vi "xiLIB - PRM_Limit.vi"(4 "PRM":T2=enum."DEVICE_NAME", 6 "Type":T1, 8 "error in (no error)":errorcluster, 9 "Ctl Refnum":refnum<vi>, 11 "xiCam In":refnum<k24>) -> (0 "error out":errorcluster, 3 "xiCam Out":refnum<k24>)   [LabVIEW 2015]
uses:
  C:/GIT/Cameras3.x/Integrations/Labview/xiLib/xiLIB_32bit/xiLIB/xiCamLib/API/x86/xiApi.NET.dll
  xiLIB_32bit/xiLIB/xiCamLib/API/x86/xiApi.NET.dll
  Typedefs/xiLIB - PRM_Type.ctl
  xiCam/PRM/PRM/PRM_v2.ctl
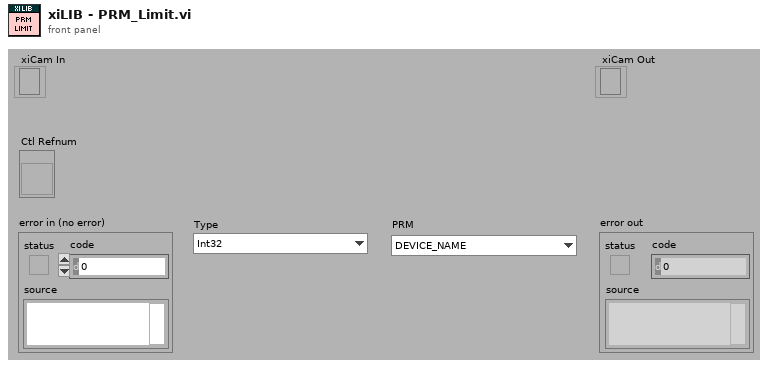
[diagram p1: front panel]
types:
  T1 = typedef "xiLIB - PRM_Type.ctl" = enum16{"Int32", "Float", "String", "DOWNSAMPLING_TYPE", "IMAGE_DATA_FORMAT", "BUFFER_POLICY", "TRG_SOURCE", "GPI", "GPO", "ACQ_TIMING_MODE", "BINNING_PATTERN", "BINNING_SELECTOR", "CMS_MODE", "COUNTER_SELECTOR", "DEBUG_LEVEL", "DECIMATION_PATTERN", "DECIMATION_SELECTOR", "GAIN_SELECTOR_TYPE", "LED_MODE", "LENS_FEATURE_SELECTOR", "LENS_MODE", "OUTPUT_DATA_PACKING_TYPE", "SENSOR_FEATURE_SELECTOR", "SHUTTER_TYPE", "TRG_SELECTOR", "TS_RST_MODE", "TS_RST_SOURCE"}
  T2 = typedef "PRM_v2.ctl" = enum16{"ACQ_BUFFER_SIZE", "ACQ_FRAME_BURST_COUNT", "ACQ_TIMING_MODE", "ACQ_TRANSPORT_BUFFER_SIZE", "AE_MAX_LIMIT", "AEAG", "AEAG_LEVEL", "API_VERSION", "AG_MAX_LIMIT", "APPLY_CMS", "AUTO_BANDWIDTH_CALCULATION", "AUTO_WB", "AVAILABLE_BANDWIDTH", "AVAILABLE_BANDWIDTH_MAX", "AVAILABLE_BANDWIDTH_MIN", "BPC", "BUFFER_POLICY", "BUFFERS_QUEUE_SIZE", "CC_MATRIX_00", "CC_MATRIX_01", "CC_MATRIX_02", "CC_MATRIX_03", "CC_MATRIX_10", "CC_MATRIX_11", "CC_MATRIX_12", "CC_MATRIX_13", "CC_MATRIX_20", "CC_MATRIX_21", "CC_MATRIX_22", "CC_MATRIX_23", "CC_MATRIX_30", "CC_MATRIX_31", "CC_MATRIX_32", "CC_MATRIX_33", "CHIP_TEMP", "CMS", "COLOR_FILTER_ARRAY", "COOLING", "DEBOUNCE_EN", "DEBOUNCE_POL", "DEBOUNCE_T0", "DEBOUNCE_T1", "DEBUG_LEVEL", "DEFAULT_CC_MATRIX", "DEVICE_INSTANCE_PATH", "DEVICE_MODEL_ID", "DEVICE_NAME", "DEVICE_SN", "DEVICE_TYPE", "DEVICE_USER_ID", "DOWNSAMPLING", "DOWNSAMPLING_MAX", "DOWNSAMPLING_MIN", "DOWNSAMPLING_TYPE", "DRV_VERSION", "EXP_PRIORITY", "EXPOSURE", "EXPOSURE_DIRECT_UPDATE", "EXPOSURE_MAX", "EXPOSURE_MIN", "FFS_FILE_NAME", "FPGA1_VERSION", "FRAMERATE", "FRAMERATE_MAX", "FRAMERATE_MIN", "FREE_FFS_SIZE", "GAIN", "GAIN_DIRECT_UPDATE", "GAIN_MAX", "GAIN_MIN", "GAMMAC", "GAMMAY", "GPI_LEVEL", "GPI_MODE", "GPI_SELECTOR", "GPI_SELECTOR_MAX", "GPI_SELECTOR_MIN", "GPO_MODE", "GPO_SELECTOR", "GPO_SELECTOR_MAX", "GPO_SELECTOR_MIN", "HDR", "HDR_T1", "HDR_T2", "HEIGHT", "HEIGHT_MAX", "HEIGHT_MIN", "HOUSE_TEMP", "IMAGE_DATA_FORMAT", "IMAGE_IS_COLOR", "INPUT_CMS_PROFILE", "IS_COOLED", "IS_DEVICE_EXIST", "KNEEPOINT1", "KNEEPOINT2", "LED_MODE", "LED_SELECTOR", "LED_SELECTOR_MAX", "LED_SELECTOR_MIN", "LIMIT_BANDWIDTH", "LIMIT_BANDWIDTH_MAX", "LIMIT_BANDWIDTH_MIN", "LUT_EN", "LUT_INDEX", "LUT_INDEX_MAX", "LUT_INDEX_MIN", "LUT_VALUE", "LUT_VALUE_MAX", "LUT_VALUE_MIN", "MANUAL_WB", "MCU1_VERSION", "MCU2_VERSION", "OFFSET_X", "OFFSET_X_MAX", "OFFSET_X_MIN", "OFFSET_Y", "OFFSET_Y_MAX", "OFFSET_Y_MIN", "OUTPUT_CMS_PROFILE", "OUTPUT_DATA_BIT_DEPTH", "OUTPUT_DATA_PACKING", "READ_FILE_FFS", "RECENT_FRAME", "SENSOR_DATA_BIT_DEPTH", "SENSOR_MODE", "SENSOR_TAPS", "SHARPNESS", "SHUTTER_TYPE", "TARGET_TEMP", "TRG_DELAY", "TRG_SELECTOR", "TRG_SOFTWARE", "TRG_SOURCE", "USED_FFS_SIZE", "WB_KB", "WB_KG", "WB_KR", "WIDTH", "WIDTH_MAX", "WIDTH_MIN", "WRITE_FILE_FFS", "ACQ_BUFFER_SIZE_UNIT", "ACQ_TRANSPORT_BUFFER_COMMIT", "AEAG_ROI_HEIGHT", "AEAG_ROI_OFFSET_X", "AEAG_ROU_OFFSET_Y", "AEAG_ROI_WIDTH", "API_CONTEXT_LIST", "BINNING_HORIZONTAL", "BINNING_SELECTOR", "BINNING_VERTICAL", "COLUMN_FPN_CORRECTION", "COUNTER_SELECTOR", "COUNTER_VALUE", "DECIMATION_HORIZONTAL", "DECIMATION_SELECTOR", "DECIMATION_VERTICAL", "DEVICE_ID", "DEVICE_LOCATION_PATH", "DEVICE_MANIFEST", "DEVICE_RESET", "DEVICE_SENS_SN", "EXPOSURE_BURST_COUNT", "FFS_ACCESS_KEY", "GAIN_SELECTOR", "HW_REVISION", "IMAGE_BLACK_LEVEL", "IMAGE_DATA_BIT_DEPTH", "IMAGE_DATA_FORMAT_RGB32_ALPHA", "IMAGE_PAYLOAD_SIZE", "LENS_APERTURE_VALUE", "LENS_FEATURE", "LENS_FEATURE_SELECTOR", "LENS_FOCAL_LENGTH", "LENS_FOCUS_DISTANCE", "LENS_FOCUS_MOVE", "LENS_FOCUS_MOVEMENT_VALUE", "LENS_MODE", "OUTPUT_DATA_PACKING_TYPE", "SENSOR_CLOCK_FREQ_HZ", "SENSOR_CLOCK_FREQ_INDEX", "SENSOR_FEATURE_SELECTOR", "SENSOR_FEATURE_VALUE", "SENSOR_OUTPUT_CHANNEL_COUNT", "TRANSPORT_PIXEL_FORMAT", "TS_RST_MODE", "TS_RST_SOURCE"}
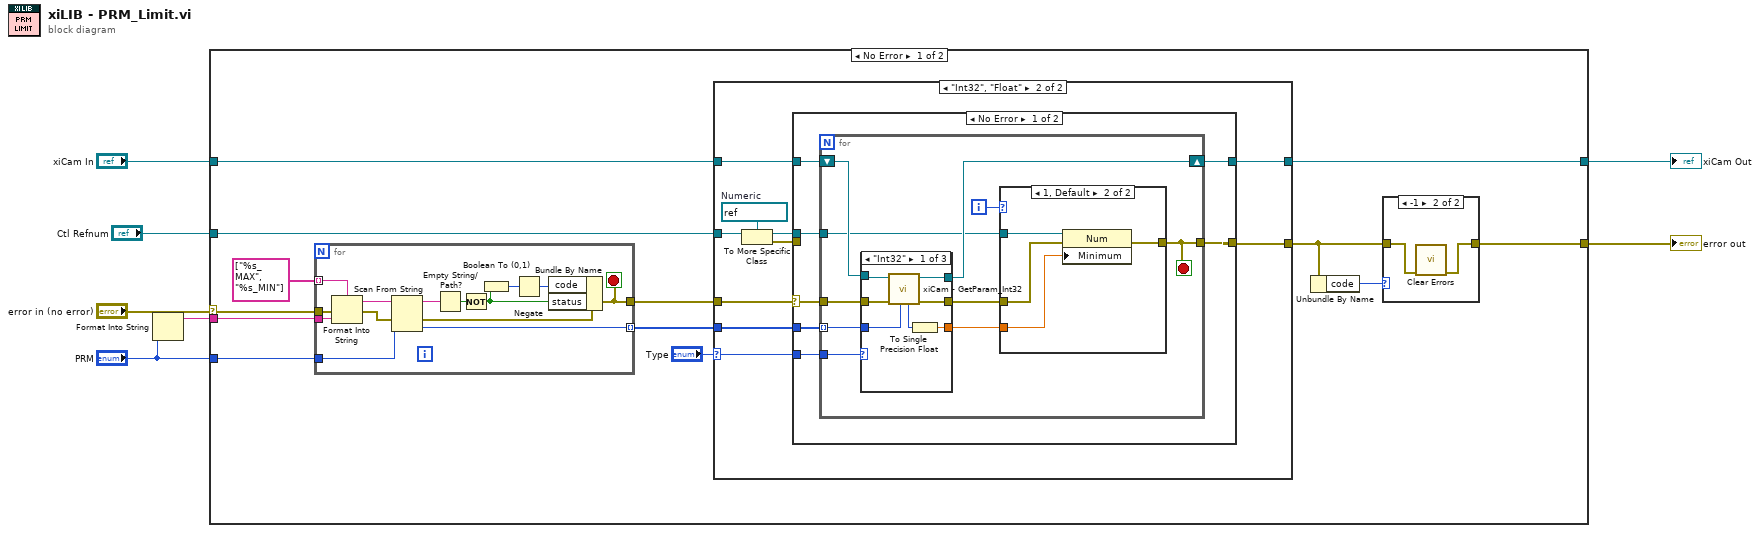
[diagram p0: block diagram]
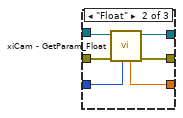
[diagram p4: hidden frame]
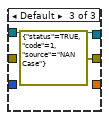
[diagram p5: hidden frame]
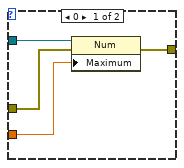
[diagram p6: hidden frame]
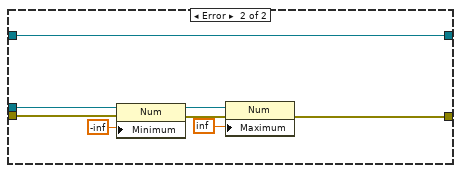
[diagram p7: hidden frame]
diagram:
  n1 = Format Into String("PRM") -> (resulting string=w3:string)  [unwired: 3 in, 1 out]
  n2 = case shown="No Error" "error in (no error)" {
    selector: "error in (no error)" -> [w18 w98]
    tunnel: "xiCam In" -> [w20 w99]
    tunnel: [w12 w99] -> w5
    tunnel: [w9 w98] -> w4
    tunnel: w3 -> [w19 _]
    tunnel: "PRM" -> [w17 _]
    tunnel: "Ctl Refnum" -> [w15 _]
    frame No Error {
      n3 = for {
        tunnel: w19 -> [w37]
        tunnel: w18 -> [w36]
        tunnel: w17 -> [w35]
        tunnel: string[] ["%s_MAX", "%s_MIN"] -> [w34] mode=indexing
        tunnel: [w28] -> w14
        tunnel: [w27] -> w13 mode=indexing
        stop <- w28 stop-if-true
        n4 = Format Into String(format string=w34, error in=w36, w37) -> (resulting string=w33:string, error out=w32:errorcluster)  [unwired: 1 in]
        n5 = Scan From String(input string=w33, error in=w32, default 1=w35) -> (remaining string=w31:string, error out=w29:errorcluster, output 1=w27:T2)  [unwired: 2 in, 1 out]
        n6 = Empty String/Path?(string/path=w31) -> (empty?=w30:bool)
        n7 = Not(x=w30) -> (.not. x?=w25:bool)
        n8 = Boolean To (0,1)(Boolean=w25) -> (0, 1=w26:i16)
        n9 = Negate(x=w26) -> (-x=w24:i16)
        n10 = Bundle By Name(cluster=w29, "code"=w24, "status"=w25) -> (w28:errorcluster)
      }
      n11 = case shown="\"Int32\", \"Float\"" "Type" {
        selector: "Type" -> [_ w40]
        tunnel: w14 -> [w38 w42]
        tunnel: w15 -> [_ w46]
        tunnel: w20 -> [w39 w49]
        tunnel: w13 -> [_ w48]
        tunnel: [w38 w44] -> w10
        tunnel: [w39 w43] -> w12
        frame Default {
        }
        frame "Int32", "Float" {
          w47 = refnum<vi> refnum  # Numeric
          n12 = To More Specific Class(target class=w47, reference=w46) -> (specific class reference=w45:refnum<vi>, error out=w41:errorcluster)  [unwired: 1 in]
          n13 = case shown="No Error" w42 {
            selector: w42 -> [w51 _]
            tunnel: w49 -> [w56 w90]
            tunnel: w48 -> [w55 _]
            tunnel: w45 -> [w54 w97]
            tunnel: [w53 w93] -> w44
            tunnel: [w52 w90] -> w43
            tunnel: w41 -> [_ w94]
            tunnel: w40 -> [w50 _]
            frame No Error {
              n14 = for {
                shift-right: [w64] -> w52
                shift-left: w56 -> [w65]
                tunnel: w55 -> [w63] mode=indexing
                tunnel: w54 -> [w61]
                tunnel: w51 -> [w66]
                tunnel: [w58] -> w53
                tunnel: w50 -> [w57]
                i -> [w62]
                stop <- w58 stop-if-true
                n15 = case shown="\"Int32\"" w57 {
                  tunnel: w66 -> [w73 w79 _]
                  tunnel: w65 -> [w72 w78 w81]
                  tunnel: [w71 w77 w81] -> w64
                  tunnel: w63 -> [w70 w76 _]
                  tunnel: [w69 w75 errorcluster {"status"=TRUE, "code"=1, "source"="NAN Case"} ("error out")] -> w60
                  tunnel: [w67 w74 _] -> w59
                  frame "Int32" {
                    n16 = call "xiCam - GetParam_Int32.vi"("PRM"=w70, "error in (no error)"=w73, "xiCam In"=w72) -> ("error out"=w69:errorcluster, "xiCam Out"=w71:refnum<k24>, "Int32_Value"=w68:i32)  [unwired: 6 in]
                    n17 = To Single Precision Float(number=w68) -> (single precision float=w67:sgl)
                  }
                  frame "Float" {
                    n18 = call "xiCam - GetParam_Float.vi"("PRM"=w76, "error in (no error)"=w79, "xiCam In"=w78) -> ("error out"=w75:errorcluster, "xiCam Out"=w77:refnum<k24>, "Float_Value"=w74:sgl)  [unwired: 6 in]
                  }
                  frame Default {
                  }
                }
                n19 = case shown="1, Default" w62 {
                  tunnel: w61 -> [w85 w89]
                  tunnel: w60 -> [w84 w88]
                  tunnel: w59 -> [w83 w87]
                  tunnel: [w82 w86] -> w58
                  frame 0 {
                    n20 = property class="Num"(reference=w85, error in=w84, "Maximum"=w83) -> (error out=w82:errorcluster)  [unwired: 1 out]
                  }
                  frame 1, Default {
                    n21 = property class="Num"(reference=w89, error in=w88, "Minimum"=w87) -> (error out=w86:errorcluster)  [unwired: 1 out]
                  }
                }
              }
            }
            frame Error {
              n22 = property class="Num"(reference=w97, error in=w94, "Minimum"=-inf) -> (reference out=w96:refnum<vi>, error out=w95:errorcluster)
              n23 = property class="Num"(reference=w96, error in=w95, "Maximum"=inf) -> (error out=w93:errorcluster)  [unwired: 1 out]
            }
          }
        }
      }
      n24 = Unbundle By Name(w10) -> ("code"=w11:i32)
      n25 = case shown="-1" w11 {
        tunnel: w10 -> [w21 w23]
        tunnel: [w21 w22] -> w9
        frame 0, Default {
        }
        frame -1 {
          n26 = call <vilib>:"Clear Errors.vi"("error in (no error)"=w23) -> ("error out"=w22:errorcluster)  [unwired: 5 in, 1 out]
        }
      }
    }
    frame Error {
    }
  }
  "error out" <- w4
  "xiCam Out" <- w5
